vi "Read Current Target.vi"(11 "BuildManager in":refnum<class "BuildManager.lvclass">) -> (2 "Current Target":string, 3 "BuildManager out":refnum<class "BuildManager.lvclass">)   [LabVIEW 2019, in "SolutionBuilder.lvlib" / "BuildManager.lvclass"]
uses:
  BuildManager.lvclass
  BuildManager.lvclass/BuildManager.ctl
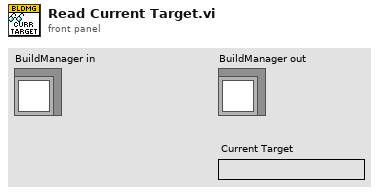
[diagram p1: front panel]
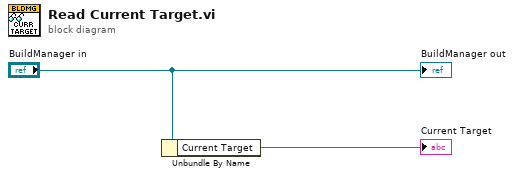
[diagram p0: block diagram]
diagram:
  n1 = Unbundle By Name("BuildManager in") -> ("Current Target"=→"Current Target":string)
  "BuildManager out" <- "BuildManager in"
